vi "Comms Loop State Controller Queue Ref.vi"(8 "error in (no error)":errorcluster) -> (0 "error out":errorcluster, 3 "queue out":refnum<queue>)   [LabVIEW 2019]
uses:
  Controls/Comms Loop State Controller Message.ctl
  Controls/Comms Loop States.ctl
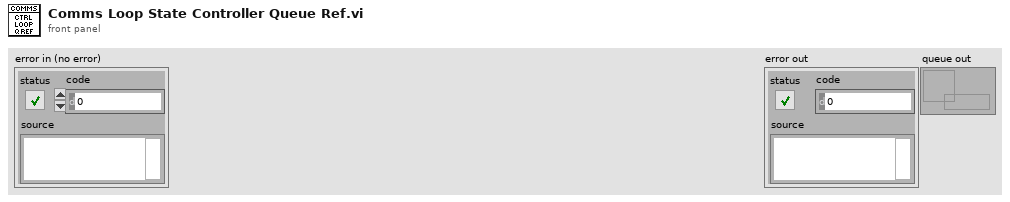
[diagram p1: front panel]
types:
  T1 = typedef "Comms Loop State Controller Message.ctl" = cluster{"Command":T2, "Data":variant}
  T2 = typedef "Comms Loop States.ctl" = enum16{"Initalise", "User Event", "HEART_BEAT", "SEND_LOG_FILE_NAME", "Clear Log File Names", "SEND_LOG_FILE_CHUNK", "SEND_LOG_FILE_SIZE", "SEND_SD_CARD_INFO", "SEND_BATTERY_INFO", "SEND_LOGGING_PERIOD", "SEND_RTC_TIME", "SEND_CURRENT_MEASUREMENTS", "ERROR_MSG", "Clear Error Messages", "Send Message", "Idle", "Sensor Connected", "Sensor Disconnected", "Set Page Displayed", "Set Connected Sensor Type", "UI: Update Sensor Type", "UI: Update Log List", "Reset Log File Transfer", "SEND_WIFI_DETAILS"}
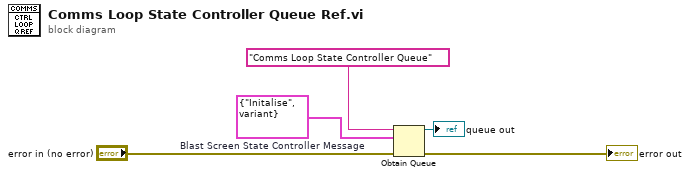
[diagram p0: block diagram]
diagram:
  w2 = T1 {"Command"=enum."Initalise", "Data"=variant}  # Blast Screen State Controller Message
  n1 = Obtain Queue(name (unnamed)="Comms Loop State Controller Queue", element data type=w2, error in (no error)="error in (no error)") -> (queue out=→"queue out":refnum<queue>, error out=→"error out":errorcluster)  [unwired: 2 in, 1 out]
